vi "Draw Arrowed Line (ARGB).vi"(4 "Tip Length (Default 0.1)":dbl=0.1, 5 "Thickness (Default: 1)":i32=1, 6 "OpenCV Line Type (Default LINE_8)":T4=enum."LINE_8", 7 "ARGB Colour":T3={"Alpha"=255, "RGB"=0}, 8 "error in (no error)":errorcluster, 9 "Pointed-to Point":T1, 10 "Start Point":T1, 11 "ARGB Image in":T2) -> (0 "error out":errorcluster, 3 "ARGB Image":T2)   [LabVIEW 2020, in "image.lvlib"]
doc: "Draw an arrowed line between two points."
uses:
  image.lvlib
  Line Type.ctl
  common/Image Point (Integer).ctl
  ARGB Image.ctl
  ARGB Colour.ctl
  c990ea83-8feb-41a3-987e-5529af170d73.vi
  <vilib>/Utility/error.llb/Error Cluster From Error Code.vi
  common/common.lvlib
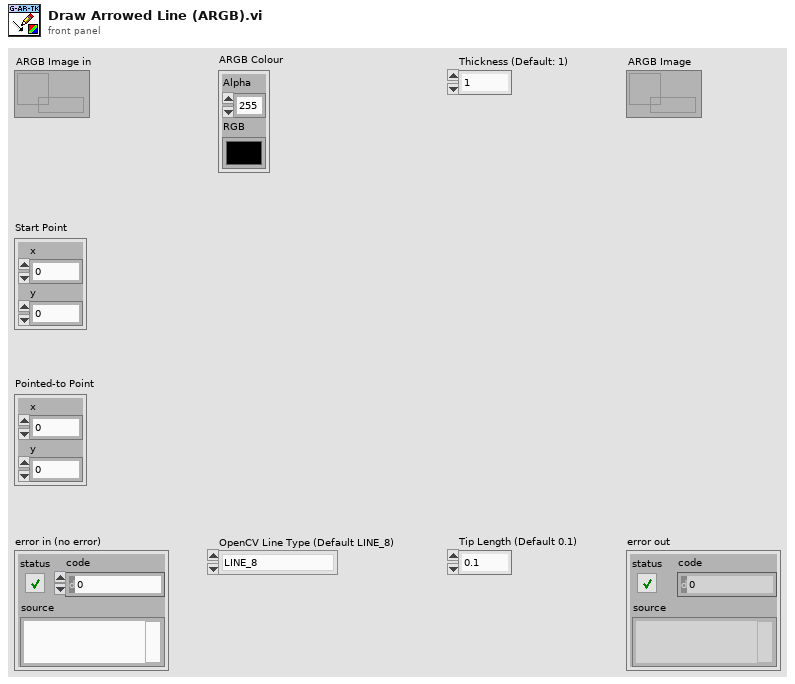
[diagram p1: front panel]
types:
  T1 = typedef "common.lvlib/Image Point (Integer).ctl" = cluster{"x":i32, "y":i32}
  T2 = typedef "image.lvlib/ARGB Image.ctl" = refnum<data-value>
  T3 = typedef "image.lvlib/ARGB Colour.ctl" = cluster{"Alpha":u8, "RGB":u32}
  T4 = typedef "image.lvlib/Line Type.ctl" = enum8{"FILLED", "LINE_4", "LINE_8", "LINE_AA"}
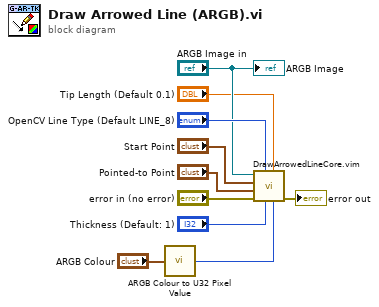
[diagram p0: block diagram]
diagram:
  n1 = call "ARGB Colour to U32 Pixel Value.vi"("ARGB Colour"="ARGB Colour") -> ("U32 Colour"=w4:u32)
  n2 = call "DrawArrowedLineCore.vim"("Colour"=w4, "Tip Length"="Tip Length (Default 0.1)", "Thickness"="Thickness (Default: 1)", "OpenCV Line Type"="OpenCV Line Type (Default LINE_8)", "error in (no error)"="error in (no error)", "Point B"="Pointed-to Point", "Point A"="Start Point", "Src"="ARGB Image in") -> ("error out"=→"error out":errorcluster)  [unwired: 3 in]
  "ARGB Image" <- "ARGB Image in"
